vi "Waveguide Model.vi"(2 "Vs (V)":dbl, 3 "Vsg (V)":dbl) -> (0 "I[Vsg] (A)":dbl, 1 "G[Vsg] (e2/h)":dbl)   [LabVIEW 2019, in "Instrument.Lockin.lvlib" / "Instrument.DAQ.lvclass"]
uses:
  Instrument.DAQ.lvclass
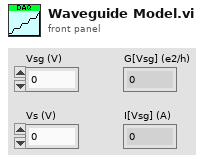
[diagram p1: front panel]
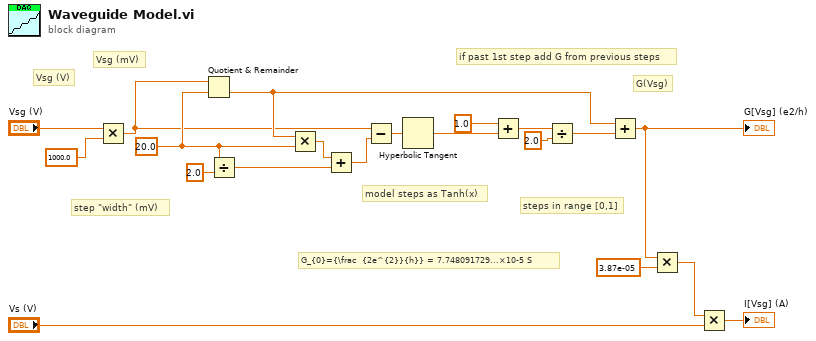
[diagram p0: block diagram]
diagram:
  w13 = 20.0 ("y")
  # "G_{0}={\\frac  {2e^{2}}{h}} = 7.748091729...×10-5 S"
  # "Vsg (mV)"
  # "if past 1st step add G from previous steps"
  # "steps in range [0,1]"
  # "model steps as Tanh(x)"
  # "step \"width\" (mV)"
  # "G(Vsg)"
  # "Vsg (V)"
  n1 = Multiply(x="Vsg (V)", y=1000.0) -> (x*y=w1:dbl)
  n2 = Quotient & Remainder(x=w1, y=w13) -> (floor(x/y)=w14:dbl)  [unwired: 1 out]
  n3 = Divide(x=w13, y=2.0) -> (x/y=w11:dbl)
  n4 = Multiply(x=w14, y=w13) -> (x*y=w8:dbl)
  n5 = Add(x=w8, y=w11) -> (x+y=w9:dbl)
  n6 = Subtract(x=w1, y=w9) -> (x-y=w3:dbl)
  n7 = Hyperbolic Tangent(1:w3) -> (0:w7:dbl)
  n8 = Add(x=1.0, y=w7) -> (x+y=w5:dbl)
  n9 = Divide(x=w5, y=2.0) -> (x/y=w2:dbl)
  n10 = Add(x=w14, y=w2) -> (x+y=w17:dbl)
  "G[Vsg] (e2/h)" <- w17
  n11 = Multiply(x=w17, y=3.87e-05) -> (x*y=w20:dbl)
  n12 = Multiply(x=w20, y="Vs (V)") -> (x*y=→"I[Vsg] (A)":dbl)
